vi "Finish.vi"   [LabVIEW 2018]
doc: "This VI is called just before exiting. It is expected to close I/O refnum, save collected data, etc."
uses:
  <vilib>/Rock Robotics/WPI/Utilities/WPI_GetSetVariantRefNum.vi
types:
  T1 = typedef "WPI_SolenoidDevRef.ctl" = cluster{"DevStatus":errorcluster, "Pneumatics Control Module":u8, "Forward Solenoid Channel":T2, "Reverse Solenoid Channel":T2}
  T2 = typedef "WPI_SolenoidChannel.ctl" = enum8{"Solenoid 0", "Solenoid 1", "Solenoid 2", "Solenoid 3", "Solenoid 4", "Solenoid 5", "Solenoid 6", "Solenoid 7", "Invalid"}
  T3 = typedef "WPI_DigitalInputDevRef.ctl" = cluster{"DevStatus":errorcluster, "DIO Channel":T4}
  T4 = typedef "FPGA_DIOChannel.ctl" = enum8{"DIO 0", "DIO 1", "DIO 2", "DIO 3", "DIO 4", "DIO 5", "DIO 6", "DIO 7", "DIO 8", "DIO 9", "DIO MXP 0", "DIO MXP 1", "DIO MXP 2", "DIO MXP 3", "DIO MXP 4", "DIO MXP 5", "DIO MXP 6", "DIO MXP 7", "DIO MXP 8", "DIO MXP 9", "DIO MXP 10", "DIO MXP 11", "DIO MXP 12", "DIO MXP 13", "DIO MXP 14", "DIO MXP 15", "SPI Port CS1", "SPI Port CS2", "SPI Port CS3", "SPI Port MISO", "SPI Port MOSI", "Invalid"}
  T5 = typedef "WPI_JoystickDevRef.ctl" = cluster{"Device":T6}
  T6 = typedef "WPI_JoystickDeviceEnum.ctl" = enum16{"USB 0", "USB 1", "USB 2", "USB 3", "USB 4", "USB 5"}
  T7 = typedef "WPI_CompressorDevRef.ctl" = cluster{"DevStatus":errorcluster, "Pneumatics Control Module":u8}
  T8 = typedef "WPI_MotorControlDeviceRef.ctl" = cluster{"DeviceStatus":errorcluster, "Type":T9, "PWM":cluster{"PWM Channel":T10, "DeadBand":T11}, "CAN":cluster{"Device Number":u8, "SetOutput VI Ref":variant, "GetOutput VI Ref":variant, "Enable VI Ref":variant, "Disable VI Ref":variant, "Data":variant}, "Invert":bool, "DIO PWM":cluster{"PWM \"Enable\" Channel":T10, "DIOChannel":T4, "PWM Rate":dbl}}
  T9 = typedef "WPI_MotorControlType.ctl" = enum16{"PWM", "CAN", "DIO PWM"}
  T10 = typedef "FPGA_DIOPWMChannel.ctl" = enum8{"PWM 0", "PWM 1", "PWM 2", "PWM 3", "PWM 4", "PWM 5", "PWM 6", "PWM 7", "PWM 8", "PWM 9", "PWM MXP 0", "PWM MXP 1", "PWM MXP 2", "PWM MXP 3", "PWM MXP 4", "PWM MXP 5", "PWM MXP 6", "PWM MXP 7", "PWM MXP 8", "PWM MXP 9", "Invalid"}
  T11 = typedef "WPI_PWMDeadband.ctl" = cluster{"Name":string, "maxPositivePwm":i32, "minPositivePwm":i32, "centerPwm":i32, "maxNegativePwm":i32, "minNegativePwm":i32, "angularRange":u16}
  T12 = typedef "ImuDevRef.ctl" = cluster{"I2CDevRef":T13, "Valid Cal File?":bool}
  T13 = typedef "WPI_I2CDevRef.ctl" = cluster{"DevStatus":errorcluster, "Device Address":u8, "Handle":i32, "I2C Bus":T14}
  T14 = typedef "i2c_bus.ctl" = enum16{"I2C On-Board", "I2C MXP", "Invalid"}
  T15 = typedef "WPI_AnalogChannelDevRef.ctl" = cluster{"DevStatus":errorcluster, "Analog Channel":T16}
  T16 = typedef "FPGA_AIChannel.ctl" = enum8{"AI 0", "AI 1", "AI 2", "AI 3", "AI MXP 0", "AI MXP 1", "AI MXP 2", "AI MXP 3", "Invalid"}
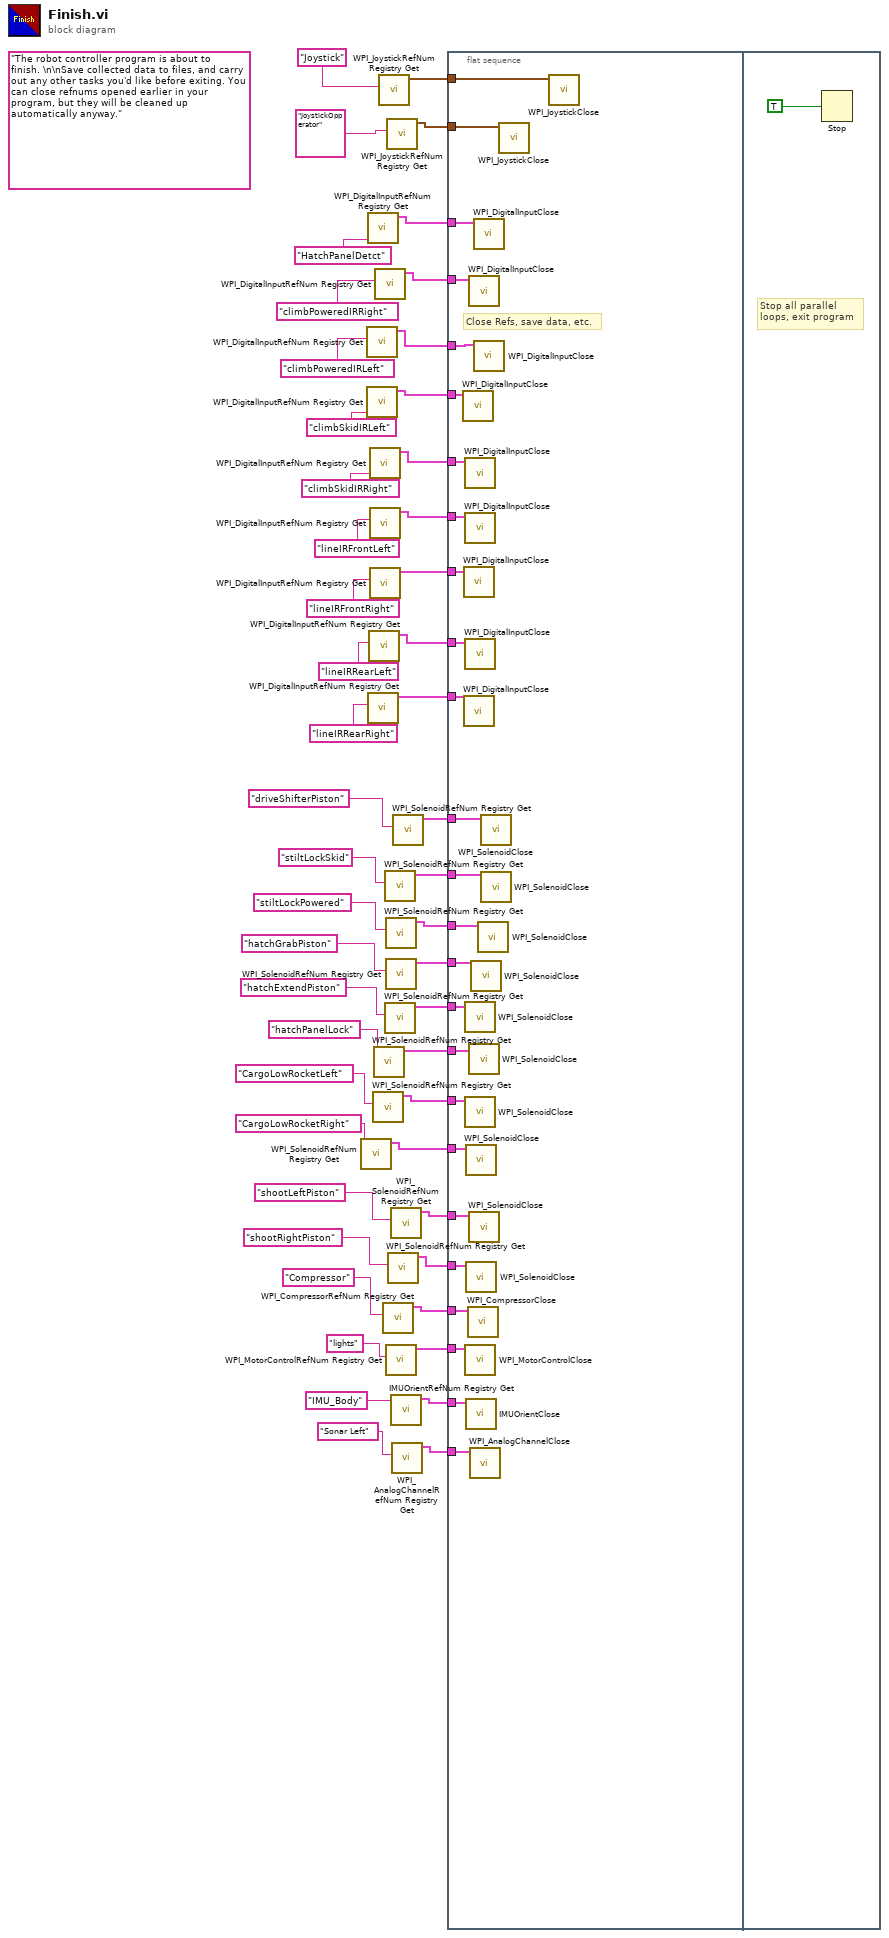
[diagram p0: block diagram]
diagram:
  (unwired) "The robot controller program is about to finish. \n\nSave collected data to files, and carry out any other tasks you'd like before exiting. You can close refnums opened earlier in your program, but they will be cleaned up automatically anyway."
  n1 = call <vilib>:"WPI_SolenoidRefNum Registry Get.vi"("refnum name"="CargoLowRocketRight") -> ("SolenoidDevRef"=w19:T1)  [unwired: 9 in, 1 out]
  n2 = call <vilib>:"WPI_DigitalInputRefNum Registry Get.vi"("refnum name"="climbPoweredIRLeft") -> ("DigitalInputDevRef"=w36:T3)  [unwired: 9 in, 1 out]
  n3 = call <vilib>:"WPI_DigitalInputRefNum Registry Get.vi"("refnum name"="climbSkidIRLeft") -> ("DigitalInputDevRef"=w35:T3)  [unwired: 9 in, 1 out]
  n4 = call <vilib>:"WPI_DigitalInputRefNum Registry Get.vi"("refnum name"="HatchPanelDetct") -> ("DigitalInputDevRef"=w38:T3)  [unwired: 9 in, 1 out]
  n5 = call <vilib>:"WPI_DigitalInputRefNum Registry Get.vi"("refnum name"="lineIRRearRight") -> ("DigitalInputDevRef"=w39:T3)  [unwired: 9 in, 1 out]
  n6 = call <vilib>:"WPI_DigitalInputRefNum Registry Get.vi"("refnum name"="lineIRRearLeft") -> ("DigitalInputDevRef"=w31:T3)  [unwired: 9 in, 1 out]
  n7 = call <vilib>:"WPI_DigitalInputRefNum Registry Get.vi"("refnum name"="climbSkidIRRight") -> ("DigitalInputDevRef"=w34:T3)  [unwired: 9 in, 1 out]
  n8 = call <vilib>:"WPI_DigitalInputRefNum Registry Get.vi"("refnum name"="lineIRFrontLeft") -> ("DigitalInputDevRef"=w33:T3)  [unwired: 9 in, 1 out]
  n9 = call <vilib>:"WPI_DigitalInputRefNum Registry Get.vi"("refnum name"="lineIRFrontRight") -> ("DigitalInputDevRef"=w32:T3)  [unwired: 9 in, 1 out]
  n10 = call <vilib>:"WPI_SolenoidRefNum Registry Get.vi"("refnum name"="CargoLowRocketLeft") -> ("SolenoidDevRef"=w18:T1)  [unwired: 9 in, 1 out]
  n11 = call <vilib>:"WPI_SolenoidRefNum Registry Get.vi"("refnum name"="hatchPanelLock") -> ("SolenoidDevRef"=w17:T1)  [unwired: 9 in, 1 out]
  n12 = call <vilib>:"WPI_DigitalInputRefNum Registry Get.vi"("refnum name"="climbPoweredIRRight") -> ("DigitalInputDevRef"=w37:T3)  [unwired: 9 in, 1 out]
  n13 = call <vilib>:"WPI_JoystickRefNum Registry Get.vi"("refnum name"="Joystick") -> ("JoystickDevRef"=w49:T5)  [unwired: 1 in, 9 out]
  n14 = call <vilib>:"WPI_CompressorRefNum Registry Get.vi"("refnum name"="Compressor") -> ("CompressorDevRef"=w9:T7)  [unwired: 9 in, 1 out]
  n15 = call <vilib>:"WPI_SolenoidRefNum Registry Get.vi"("refnum name"="stiltLockSkid") -> ("SolenoidDevRef"=w21:T1)  [unwired: 9 in, 1 out]
  n16 = call <vilib>:"WPI_SolenoidRefNum Registry Get.vi"("refnum name"="hatchExtendPiston") -> ("SolenoidDevRef"=w15:T1)  [unwired: 9 in, 1 out]
  n17 = call <vilib>:"WPI_SolenoidRefNum Registry Get.vi"("refnum name"="stiltLockPowered") -> ("SolenoidDevRef"=w20:T1)  [unwired: 9 in, 1 out]
  n18 = call <vilib>:"WPI_SolenoidRefNum Registry Get.vi"("refnum name"="hatchGrabPiston") -> ("SolenoidDevRef"=w16:T1)  [unwired: 9 in, 1 out]
  n19 = call <vilib>:"WPI_MotorControlRefNum Registry Get.vi"("refnum name"="lights") -> ("MotorControlDevRef"=w7:T8)  [unwired: 9 in, 1 out]
  n20 = call <vilib>:"WPI_JoystickRefNum Registry Get.vi"("refnum name"="JoystickOpperator") -> ("JoystickDevRef"=w3:T5)  [unwired: 9 in, 1 out]
  n21 = call <vilib>:"WPI_SolenoidRefNum Registry Get.vi"("refnum name"="shootRightPiston") -> ("SolenoidDevRef"=w11:T1)  [unwired: 9 in, 1 out]
  n22 = call <vilib>:"WPI_SolenoidRefNum Registry Get.vi"("refnum name"="shootLeftPiston") -> ("SolenoidDevRef"=w12:T1)  [unwired: 9 in, 1 out]
  n23 = call <userlib>:"IMUOrientRefNum Registry Get.vi"("refnum name"="IMU_Body") -> ("IMUDevRef out"=w5:T12)  [unwired: 9 in, 1 out]
  n24 = call <vilib>:"WPI_AnalogChannelRefNum Registry Get.vi"("refnum name"="Sonar Left") -> ("AIDeviceRef"=w1:T15)  [unwired: 9 in, 1 out]
  n25 = call <vilib>:"WPI_SolenoidRefNum Registry Get.vi"("refnum name"="driveShifterPiston") -> ("SolenoidDevRef"=w22:T1)  [unwired: 9 in, 1 out]
  n26 = flat-sequence {
    tunnel: w49 -> [w75]
    tunnel: w39 -> [w74]
    tunnel: w38 -> [w73]
    tunnel: w37 -> [w72]
    tunnel: w36 -> [w71]
    tunnel: w35 -> [w70]
    tunnel: w34 -> [w69]
    tunnel: w33 -> [w68]
    tunnel: w32 -> [w67]
    tunnel: w31 -> [w66]
    tunnel: w22 -> [w65]
    tunnel: w21 -> [w64]
    tunnel: w20 -> [w63]
    tunnel: w19 -> [w62]
    tunnel: w18 -> [w61]
    tunnel: w17 -> [w60]
    tunnel: w16 -> [w59]
    tunnel: w15 -> [w58]
    tunnel: w12 -> [w57]
    tunnel: w11 -> [w56]
    tunnel: w9 -> [w55]
    tunnel: w7 -> [w54]
    tunnel: w5 -> [w53]
    tunnel: w3 -> [w52]
    tunnel: w1 -> [w51]
    frame #0 {
      # "Close Refs, save data, etc."
      n27 = call <vilib>:"WPI_DigitalInputClose.vi"("DigitalInputDevRef"=w70) -> ()  [unwired: 10 in, 1 out]
      n28 = call <vilib>:"WPI_DigitalInputClose.vi"("DigitalInputDevRef"=w67) -> ()  [unwired: 10 in, 1 out]
      n29 = call <vilib>:"WPI_DigitalInputClose.vi"("DigitalInputDevRef"=w74) -> ()  [unwired: 10 in, 1 out]
      n30 = call <vilib>:"WPI_DigitalInputClose.vi"("DigitalInputDevRef"=w69) -> ()  [unwired: 10 in, 1 out]
      n31 = call <vilib>:"WPI_DigitalInputClose.vi"("DigitalInputDevRef"=w68) -> ()  [unwired: 10 in, 1 out]
      n32 = call <vilib>:"WPI_DigitalInputClose.vi"("DigitalInputDevRef"=w66) -> ()  [unwired: 10 in, 1 out]
      n33 = call <vilib>:"WPI_SolenoidClose.vi"("SolenoidDevRef"=w58) -> ()  [unwired: 10 in, 1 out]
      n34 = call <vilib>:"WPI_SolenoidClose.vi"("SolenoidDevRef"=w61) -> ()  [unwired: 10 in, 1 out]
      n35 = call <vilib>:"WPI_MotorControlClose.vi"("MotorControlDevRef"=w54) -> ()  [unwired: 10 in, 1 out]
      n36 = call <vilib>:"WPI_SolenoidClose.vi"("SolenoidDevRef"=w62) -> ()  [unwired: 10 in, 1 out]
      n37 = call <vilib>:"WPI_SolenoidClose.vi"("SolenoidDevRef"=w56) -> ()  [unwired: 10 in, 1 out]
      n38 = call <userlib>:"IMUOrientClose.vi"("IMU Dev Ref"=w53) -> ()  [unwired: 11 in]
      n39 = call <vilib>:"WPI_CompressorClose.vi"("CompressorDevRef"=w55) -> ()  [unwired: 10 in, 1 out]
      n40 = call <vilib>:"WPI_DigitalInputClose.vi"("DigitalInputDevRef"=w72) -> ()  [unwired: 10 in, 1 out]
      n41 = call <vilib>:"WPI_SolenoidClose.vi"("SolenoidDevRef"=w60) -> ()  [unwired: 10 in, 1 out]
      n42 = call <vilib>:"WPI_SolenoidClose.vi"("SolenoidDevRef"=w57) -> ()  [unwired: 10 in, 1 out]
      n43 = call <vilib>:"WPI_AnalogChannelClose.vi"("AIDeviceRef"=w51) -> ()  [unwired: 10 in, 1 out]
      n44 = call <vilib>:"WPI_SolenoidClose.vi"("SolenoidDevRef"=w59) -> ()  [unwired: 10 in, 1 out]
      n45 = call <vilib>:"WPI_DigitalInputClose.vi"("DigitalInputDevRef"=w73) -> ()  [unwired: 10 in, 1 out]
      n46 = call <vilib>:"WPI_DigitalInputClose.vi"("DigitalInputDevRef"=w71) -> ()  [unwired: 10 in, 1 out]
      n47 = call <vilib>:"WPI_SolenoidClose.vi"("SolenoidDevRef"=w63) -> ()  [unwired: 10 in, 1 out]
      n48 = call <vilib>:"WPI_SolenoidClose.vi"("SolenoidDevRef"=w65) -> ()  [unwired: 10 in, 1 out]
      n49 = call <vilib>:"WPI_SolenoidClose.vi"("SolenoidDevRef"=w64) -> ()  [unwired: 10 in, 1 out]
      n50 = call <vilib>:"WPI_JoystickClose.vi"("JoystickDevRef"=w52) -> ()  [unwired: 11 in]
      n51 = call <vilib>:"WPI_JoystickClose.vi"("JoystickDevRef"=w75) -> ()  [unwired: 11 out]
    }
    frame #1 {
      # "Stop all parallel\nloops, exit program"
      n52 = Stop(stop? (T)=TRUE ("Quit")) -> ()
    }
  }
